vi "Normalize dBm Array.vi"(4 "Input Array, dBm":dbl[](array[numeric]) format="%.2f") -> (1 "Normalized Array, delta dB":dbl[](array[numeric]) format="%.2f")   [LabVIEW 2011]
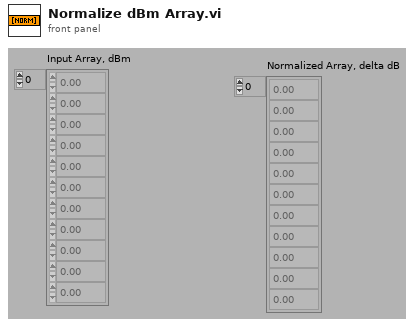
[diagram p1: front panel]
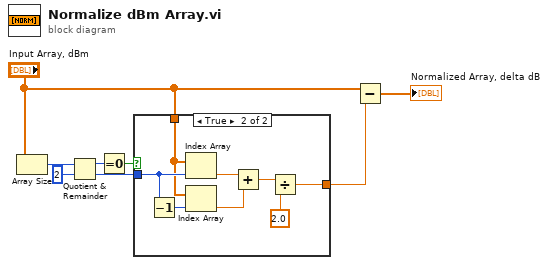
[diagram p0: block diagram]
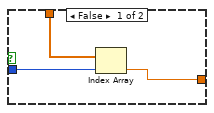
[diagram p2: hidden frame]
diagram:
  n1 = Array Size(array="Input Array, dBm") -> (size(s)=w8:i32)
  n2 = Quotient & Remainder(x=w8, y=2) -> (x-y*floor(x/y)=w5:i32, floor(x/y)=w4:i32)
  n3 = Equal To 0?(x=w5) -> (x = 0?=w1:bool)
  n4 = case shown="True" w1 {
    tunnel: w4 -> [w10 w19]
    tunnel: "Input Array, dBm" -> [w11 w16]
    tunnel: [w9 w12] -> w2
    frame False {
      n5 = Index Array(array=w11, index=w10) -> (element=w9:dbl)
    }
    frame True {
      n6 = Decrement(x=w19) -> (x-1=w18:i32)
      n7 = Index Array(array=w16, index=w19) -> (element=w15:dbl)
      n8 = Index Array(array=w16, index=w18) -> (element=w17:dbl)
      n9 = Add(x=w15, y=w17) -> (x+y=w14:dbl)
      n10 = Divide(x=w14, y=2.0) -> (x/y=w12:dbl)
    }
  }
  n11 = Subtract(x="Input Array, dBm", y=w2) -> (x-y=→"Normalized Array, delta dB":dbl[])
